vi "Buffer Data.vi"(8 "error in (no error)":errorcluster, 9 "Time Stamp (Now)":timestamp, 10 "Data":dbl[](array[numeric]), 11 "Data Buffer in":refnum<class "Data Buffer.lvclass">) -> (0 "error out":errorcluster, 3 "Data Buffer out":refnum<class "Data Buffer.lvclass">)   [LabVIEW 2020, in "VolatusData.lvlib" / "Data Buffer.lvclass"]
uses:
  Data Buffer.lvclass
  Data Buffer.lvclass/Data Buffer.ctl
  VolatusData.lvlib
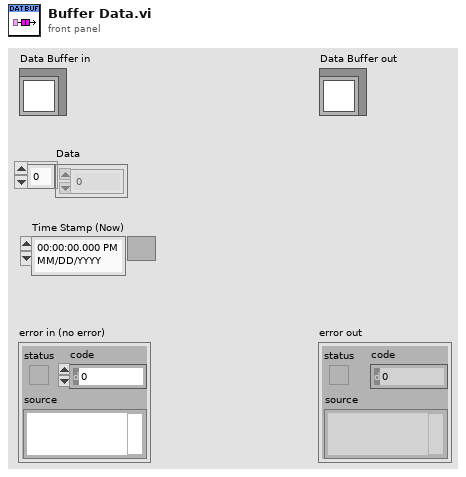
[diagram p1: front panel]
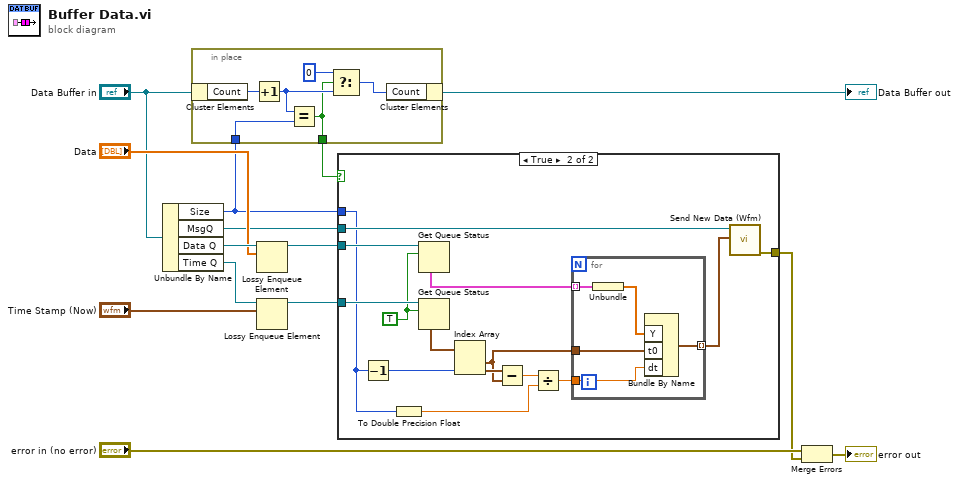
[diagram p0: block diagram]
diagram:
  n1 = Unbundle By Name("Data Buffer in") -> ("Size"=w1:i32, "MsgQ"=w6:refnum<class "MessageQ.lvclass">, "Data Q"=w13:refnum<queue>, "Time Q"=w12:refnum<queue>)
  n2 = in-place {
    in-place-border: w1 -> [w19]
    in-place-border: [w17] -> w7
    n3 = in-place-cluster #1("Data Buffer in") -> ("Count"=w20:i32)
    n4 = Increment(x=w20) -> (x+1=w18:i32)
    n5 = Equal?(x=w18, y=w19) -> (x = y?=w17:bool)
    n6 = Select(t=0, s=w17, f=w18) -> (s? t:f=w15:i32)
    n7 = in-place-cluster #1("Count"=w15) -> (→"Data Buffer out":refnum<class "Data Buffer.lvclass">)
  }
  n8 = Lossy Enqueue Element(queue=w13, element="Data") -> (queue out=w5:refnum<queue>)  [unwired: 1 in, 3 out]
  n9 = Lossy Enqueue Element(queue=w12, element="Time Stamp (Now)") -> (queue out=w4:refnum<queue>)  [unwired: 1 in, 3 out]
  n10 = case shown="True" w7 {
    tunnel: w6 -> [_ w33]
    tunnel: w5 -> [_ w35]
    tunnel: w4 -> [_ w34]
    tunnel: [_ w32] -> w2
    tunnel: w1 -> [_ w29]
    frame False {
    }
    frame True {
      w31 = TRUE ("return elements? (F)")
      n11 = Decrement(x=w29) -> (x-1=w30:i32)
      n12 = To Double Precision Float(number=w29) -> (double precision float=w27:dbl)
      n13 = Get Queue Status(queue=w35, return elements? (F)=w31) -> (elements=w26:cluster{dbl[]}[])  [unwired: 1 in, 7 out]
      n14 = Get Queue Status(queue=w34, return elements? (F)=w31) -> (elements=w24:timestamp[])  [unwired: 1 in, 7 out]
      n15 = Index Array(array=w24, index #2=w30) -> (element #1=w22:timestamp, element #2=w23:timestamp)  [unwired: 1 in]
      n16 = Subtract(x=w23, y=w22) -> (x-y=w28:dbl)
      n17 = Divide(x=w28, y=w27) -> (x/y=w25:dbl)
      n18 = for {
        tunnel: w26 -> [w40] mode=indexing
        tunnel: w25 -> [w37]
        tunnel: w22 -> [w38]
        tunnel: [w36] -> w21 mode=indexing
        n19 = Unbundle(w40) -> (w39:dbl[])
        n20 = Bundle By Name("Y"=w39, "t0"=w38, "dt"=w37) -> (w36:waveform(dbl))  [unwired: 1 in]
      }
      n21 = call "Send New Data (Wfm).vi"("Channels"=w21, "MessageQ"=w33) -> ("error out"=w32:errorcluster)  [unwired: 9 in]
    }
  }
  n22 = Merge Errors("error in (no error)", w2) -> (→"error out":errorcluster)
